vi "Dynamixel Unit Scale.vi"(3 "Model Number":u32, 4 "Data in":u32, 5 "Function":T1) -> (1 "Data out":u32)   [LabVIEW 2022 SP3]
uses:
  Dynamixel Commands.ctl
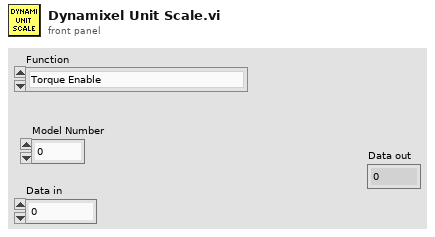
[diagram p1: front panel]
types:
  T1 = typedef "Dynamixel Commands.ctl" = enum16{"Torque Enable", "Present Position", "Threshold", "Max Position Limit", "Acceleration Profile", "Velocity Profile", "Goal Position", "Position Proportional Gain", "Position Integral Gain", "Position Differential Gain ", "Shutdown", "Write Operating Mode", "Read Operating Mode"}
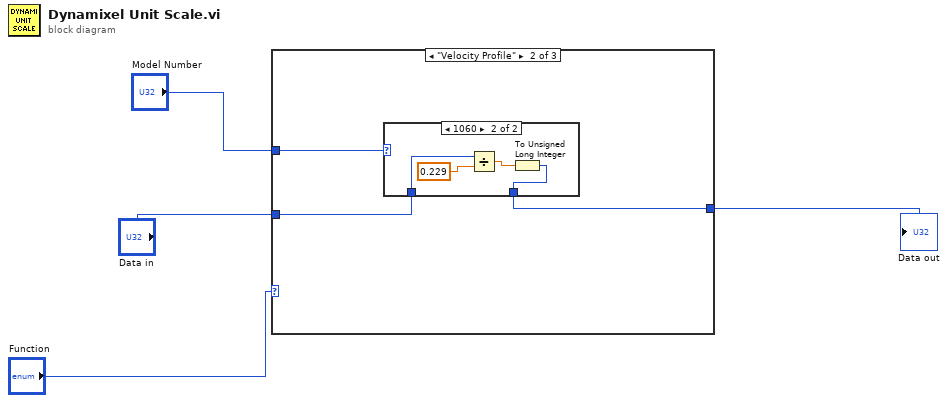
[diagram p0: block diagram]
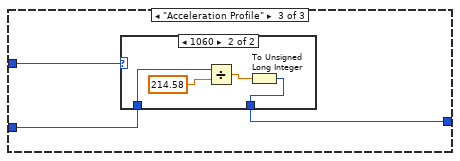
[diagram p4: hidden frame]
diagram:
  n1 = case shown="\"Velocity Profile\"" "Function" {
    tunnel: "Model Number" -> [_ w8 w16]
    tunnel: "Data in" -> [w5 w7 w15]
    tunnel: [w5 w6 w14] -> w2
    frame Default {
    }
    frame "Velocity Profile" {
      n2 = case shown="1060" w8 {
        tunnel: [w9 w10] -> w6
        tunnel: w7 -> [w9 w13]
        frame Default {
        }
        frame 1060 {
          n3 = Divide(x=w13, y=0.229) -> (x/y=w11:dbl)
          n4 = To Unsigned Long Integer(number=w11) -> (unsigned 32bit integer=w10:u32)
        }
      }
    }
    frame "Acceleration Profile" {
      n5 = case shown="1060" w16 {
        tunnel: [w17 w18] -> w14
        tunnel: w15 -> [w17 w21]
        frame Default {
        }
        frame 1060 {
          n6 = Divide(x=w21, y=214.58) -> (x/y=w19:dbl)
          n7 = To Unsigned Long Integer(number=w19) -> (unsigned 32bit integer=w18:u32)
        }
      }
    }
  }
  "Data out" <- w2
